vi "ModuleNRSD.vi"(10 "JQMHStartup.lvclass":refnum<class "JQMHStartup.lvclass">, 11 "JQMHCore in":refnum<class "JQMHModule.lvclass">) -> ()   [LabVIEW 2024, in "JQMHModule.lvclass"]
uses:
  JQMHModule.lvclass
  JQMHStartup/JQMHStartup.lvclass
  JQMHModule.lvclass/JQMHModule.ctl
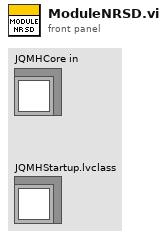
[diagram p1: front panel]
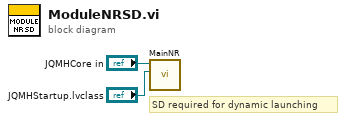
[diagram p0: block diagram]
diagram:
  # "SD required for dynamic launching"
  n1 = call-dynamic "MainNR.vi"("JQMHStartup.lvclass"="JQMHStartup.lvclass", "JQMHCore in"="JQMHCore in") -> ()  [unwired: 10 in]
